vi "Get Strings from Ref.vi"(8 "error in (no error)":errorcluster, 9 "Label Prefix":string, 10 "GObj Refnum in":refnum<vi>, 11 "WaveformGraph in":refnum<class "WaveformChart.lvclass">) -> (0 "error out":errorcluster, 1 "Valid?":bool, 2 "GObj Refnum out":refnum<vi>, 3 "WaveformGraph out":refnum<class "WaveformChart.lvclass">, 4 "GObj Name":string)   [LabVIEW 2013, in "SET Project Data.lvlib" / "WaveformChart.lvclass"]
uses:
  WaveformChart.lvclass
  GraphChart/GraphChart.lvclass
  GObject/GObject.lvclass/GObject.ctl
  GObject/Write UID.vi
  SET Project Data.lvlib
  GObject/GObject.lvclass
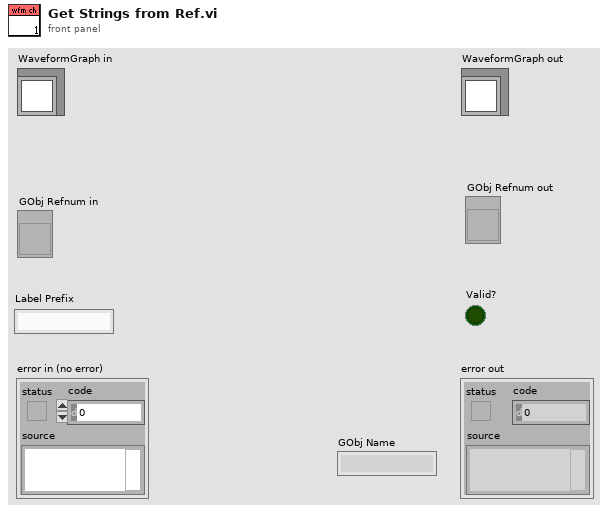
[diagram p1: front panel]
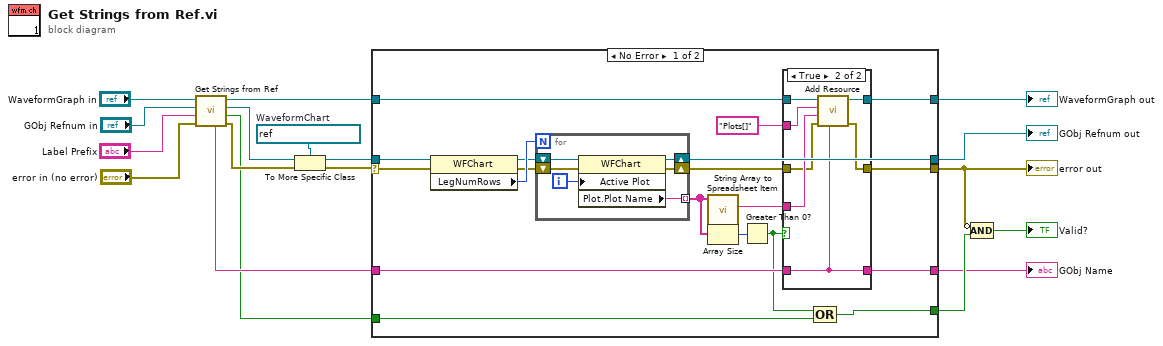
[diagram p0: block diagram]
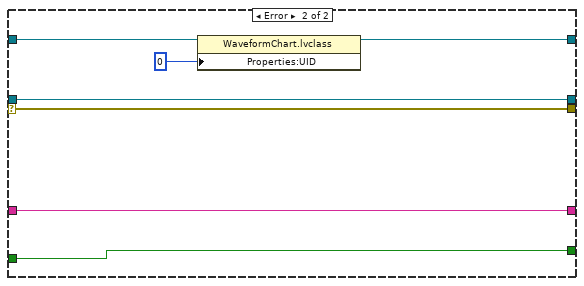
[diagram p3: hidden frame]
diagram:
  w13 = refnum<vi> refnum  # WaveformChart
  n1 = call-parent "Get Strings from Ref.vi"("error in (no error)"="error in (no error)", "Label Prefix"="Label Prefix", "GObj Refnum in"="GObj Refnum in", "GraphChart in"="WaveformGraph in") -> ("error out"=w9:errorcluster, "Valid?"=w7:bool, "GObj Refnum out"=w10:refnum<vi>, "GraphChart out"=w11:refnum<class "WaveformChart.lvclass">, "GObj Name"=w8:string)  [unwired: 3 in]
  n2 = To More Specific Class(target class=w13, reference=w10, error in=w9) -> (specific class reference=w6:refnum<vi>, error out=w12:errorcluster)
  n3 = case shown="No Error" w12 {
    selector: w12 -> [w25 w59]
    tunnel: w6 -> [w26 w60]
    tunnel: w11 -> [w36 w58]
    tunnel: [w21 w56] -> w5
    tunnel: [w20 w59] -> w2
    tunnel: [w22 w60] -> w4
    tunnel: w8 -> [w33 w55]
    tunnel: w7 -> [w31 w54]
    tunnel: [w19 w55] -> w1
    tunnel: [w30 w54] -> w14
    frame No Error {
      n4 = property class="WFChart"(reference=w26, error in=w25) -> (reference out=w28:refnum<vi>, error out=w27:errorcluster, "LegNumRows"=w29:u32)
      n5 = for {
        N: w29 -> [_]
        shift-right: [w42] -> w22
        shift-left: w28 -> [w43]
        shift-right: [w39] -> w24
        shift-left: w27 -> [w40]
        tunnel: [w38] -> w23 mode=indexing
        i -> [w41]
        n6 = property class="WFChart"(reference=w43, error in=w40, "Active Plot"=w41) -> (reference out=w42:refnum<vi>, error out=w39:errorcluster, "Plot.Plot Name"=w38:string)
      }
      n7 = call "String Array to Spreadsheet Item.vi"("Strings [] (ASCII)"=w23) -> ("Spreadsheet Item (ASCII)"=w34:string)  [unwired: 10 in]
      n8 = Array Size(array=w23) -> (size(s)=w37:i32)
      n9 = Greater Than 0?(x=w37) -> (x > 0?=w32:bool)
      n10 = case shown="True" w32 {
        tunnel: w36 -> [w46 w53]
        tunnel: [w46 w52] -> w21
        tunnel: w33 -> [w45 w49]
        tunnel: w34 -> [_ w51]
        tunnel: "Plots[]" -> [_ w50]
        tunnel: [w45 w49] -> w19
        tunnel: w24 -> [w44 w48]
        tunnel: [w44 w47] -> w20
        frame False {
        }
        frame True {
          n11 = call "Add Resource.vi"("TagPrefix"=w49, "error in (no error)"=w48, "ItemText"=w51, "ItemName"=w50, "GObject in"=w53) -> ("error out"=w47:errorcluster, "GObject out"=w52:refnum<class "WaveformChart.lvclass">)  [unwired: 5 in]
        }
      }
      n12 = Compound Arithmetic op=OR(w32, w31) -> (w30:bool)
    }
    frame Error {
      n13 = property class="WaveformChart.lvclass"(reference=w58, "Properties:UID"=0 ("UID")) -> (reference out=w56:refnum<class "WaveformChart.lvclass">)  [unwired: 1 in, 1 out]
    }
  }
  "error out" <- w2
  "WaveformGraph out" <- w5
  "GObj Refnum out" <- w4
  "GObj Name" <- w1
  n14 = Compound Arithmetic op=AND(invert w2, w14) -> (→"Valid?":bool)
